vi "Autonomous Time Elapsed.vi"(8 "Match Start Time":u32, 10 "State in":T1, 11 "State Start Time":u32) -> (0 "State Time Elapsed":u32, 2 "State out":T1, 3 "State Start Time out":u32)   [LabVIEW 2013]
uses:
  Auto Two Ball States.ctl
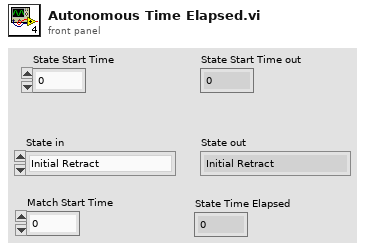
[diagram p1: front panel]
types:
  T1 = typedef "Auto Two Ball States.ctl" = enum16{"Initial Retract", "Initial Retract Wait", "First Shot: Wait for ball", "First Shot: Shoot", "Second Shot: Wait for Arm", "Grab Second Ball", "Grab Second Ball Wait", "Second Shot: Wait for ball", "Second Shot: Shoot", "Drive Forward", "Finish"}
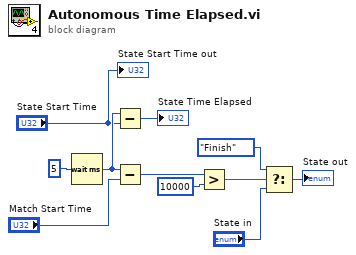
[diagram p0: block diagram]
diagram:
  n1 = Wait (ms)(milliseconds to wait=u32 5) -> (millisecond timer value=w9:u32)
  n2 = Subtract(x=w9, y="State Start Time") -> (x-y=→"State Time Elapsed":u32)
  n3 = Subtract(x=w9, y="Match Start Time") -> (x-y=w10:u32)
  n4 = Greater?(x=w10, y=u32 10000) -> (0:w4:bool)
  n5 = Select(t=Auto_Two_Ball_States."Finish", s=w4, f="State in") -> (s? t:f=→"State out":T1)
  "State Start Time out" <- "State Start Time"
